vi "Acceleration.vi"(0 "Joystick Input":dbl, 1 "MaxSpeed":dbl, 2 "Stop":bool) -> (7 "Speed":dbl)   [LabVIEW 2013]
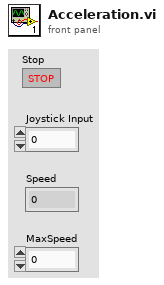
[diagram p1: front panel]
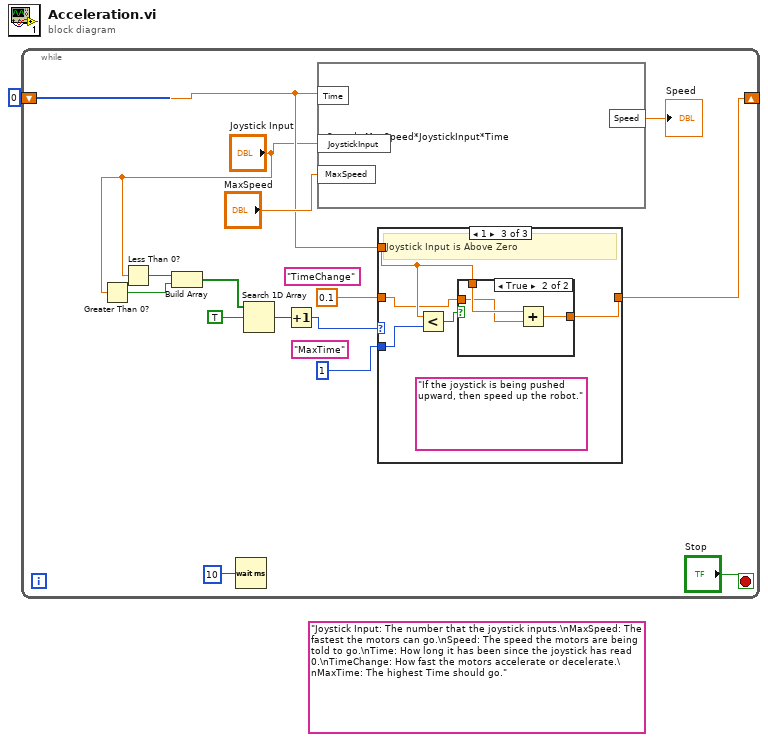
[diagram p0: block diagram]
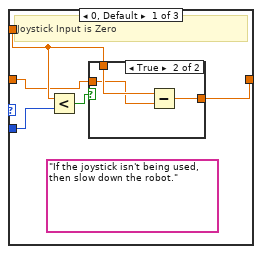
[diagram p2: hidden frame]
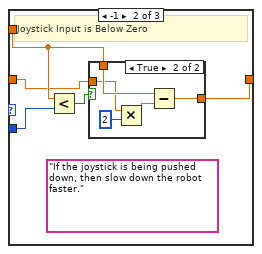
[diagram p4: hidden frame]
diagram:
  (unwired) "Joystick Input: The number that the joystick inputs.\nMaxSpeed: The fastest the motors can go.\nSpeed: The speed the motors are being told to go.\nTime: How long it has been since the joystick has read 0.\nTimeChange: How fast the motors accelerate or decelerate.\nMaxTime: The highest Time should go."
  n1 = while {
    shift-right: [w12] -> _
    shift-left: 0 -> [w11]
    stop <- "Stop" stop-if-true
    (unwired) "MaxTime"
    (unwired) "TimeChange"
    n2 = Greater Than 0?(x="Joystick Input") -> (x > 0?=w6:bool)
    n3 = Less Than 0?(x="Joystick Input") -> (x < 0?=w7:bool)
    n4 = Build Array(w7, w6) -> (w5:bool[])
    n5 = Wait (ms)(milliseconds to wait=10) -> ()  [unwired: 1 out]
    n6 = Search 1D Array(1D array=w5, element=TRUE) -> (index of element=w4:i32)  [unwired: 1 in]
    n7 = Increment(x=w4) -> (x+1=w3:i32)
    n8 = formula code="Speed=MaxSpeed*JoystickInput*Time"("Time"=w11, "JoystickInput"="Joystick Input", "MaxSpeed"="MaxSpeed") -> ("Speed"=→"Speed":dbl)
    n9 = case shown="1" w3 {
      tunnel: w11 -> [w19 w28 w39]
      tunnel: [w20 w29 w40] -> w12
      tunnel: 0.1 -> [w18 w27 w38]
      tunnel: 1 -> [w21 w30 w41]
      frame 0, Default {
        (unwired) "If the joystick isn't being used, then slow down the robot."
        # "Joystick Input is Zero"
        n10 = Less?(x=w19, y=w21) -> (x < y?=w17:bool)
        n11 = case shown="True" w17 {
          tunnel: [w22 w25] -> w20
          tunnel: w19 -> [w22 w24]
          tunnel: w18 -> [_ w23]
          frame False {
          }
          frame True {
            n12 = Subtract(x=w24, y=w23) -> (x-y=w25:dbl)
          }
        }
      }
      frame -1 {
        (unwired) "If the joystick is being pushed down, then slow down the robot faster."
        # "Joystick Input is Below Zero"
        n13 = Less?(x=w28, y=w30) -> (x < y?=w26:bool)
        n14 = case shown="True" w26 {
          tunnel: [w31 w36] -> w29
          tunnel: w28 -> [w31 w35]
          tunnel: w27 -> [_ w33]
          frame False {
          }
          frame True {
            n15 = Multiply(x=w33, y=2) -> (x*y=w34:dbl)
            n16 = Subtract(x=w35, y=w34) -> (x-y=w36:dbl)
          }
        }
      }
      frame 1 {
        (unwired) "If the joystick is being pushed upward, then speed up the robot."
        # "Joystick Input is Above Zero"
        n17 = Less?(x=w39, y=w41) -> (x < y?=w37:bool)
        n18 = case shown="True" w37 {
          tunnel: [w42 w45] -> w40
          tunnel: w39 -> [w42 w44]
          tunnel: w38 -> [_ w43]
          frame False {
          }
          frame True {
            n19 = Add(x=w44, y=w43) -> (x+y=w45:dbl)
          }
        }
      }
    }
  }
